vi "Create Cross Array.vi"() -> ()   [LabVIEW 2014]
uses:
  Slicer/LVslicer/Slice/TypeDefs/PowerSpeed.ctl
  Slicer/LVslicer/Slice/TypeDefs/PathSupreme.ctl
  Slicer/LVslicer/Slice/OverhangParam/PSup2SCAN/Sub/VelocityProfile.ctl
  Slicer/LVslicer/Slice/OverhangParam/PSup2SCAN/Sub/PathCut.ctl
  Slicer/LVslicer/Slice/OverhangParam/PSup2SCAN/Sub/Segment.ctl
  Slicer_11-28/LVslicer/Slice/TypeDefs/Point3D.ctl
  <vilib>/picture/3D Picture Control/Object/Create Object (name).vi
  <vilib>/picture/3D Picture Control/NI_3D Picture Control.lvlib
panel:
  out "Scale":cluster{dbl, dbl, dbl}
  in  "Spacing(mm)":dbl
  in  "Plate \nDiameter (mm)":dbl
  out "Stoped":bool
  in  "HighPower":dbl=500.0
  in  "Display":T1={"Mode"=enum."Inherit Value", "PointSize"=1.0, "LineWidth"=1.0}
  out "3D Picture":refnum<vi>(3d-picture)
  out "PathSupreme":T2
  in  "stop":bool
  in  "Create Array":bool
  in  "Create Cross":bool
  in  "Beam Width":dbl
  in  "# of Layers":dbl
  in  "Cross X dimension\n(cross is square)":dbl
  in  "HatchPower":T6={"Power"=300.0, "Mark Speed"=400.0, "Jump Speed"=1000.0}
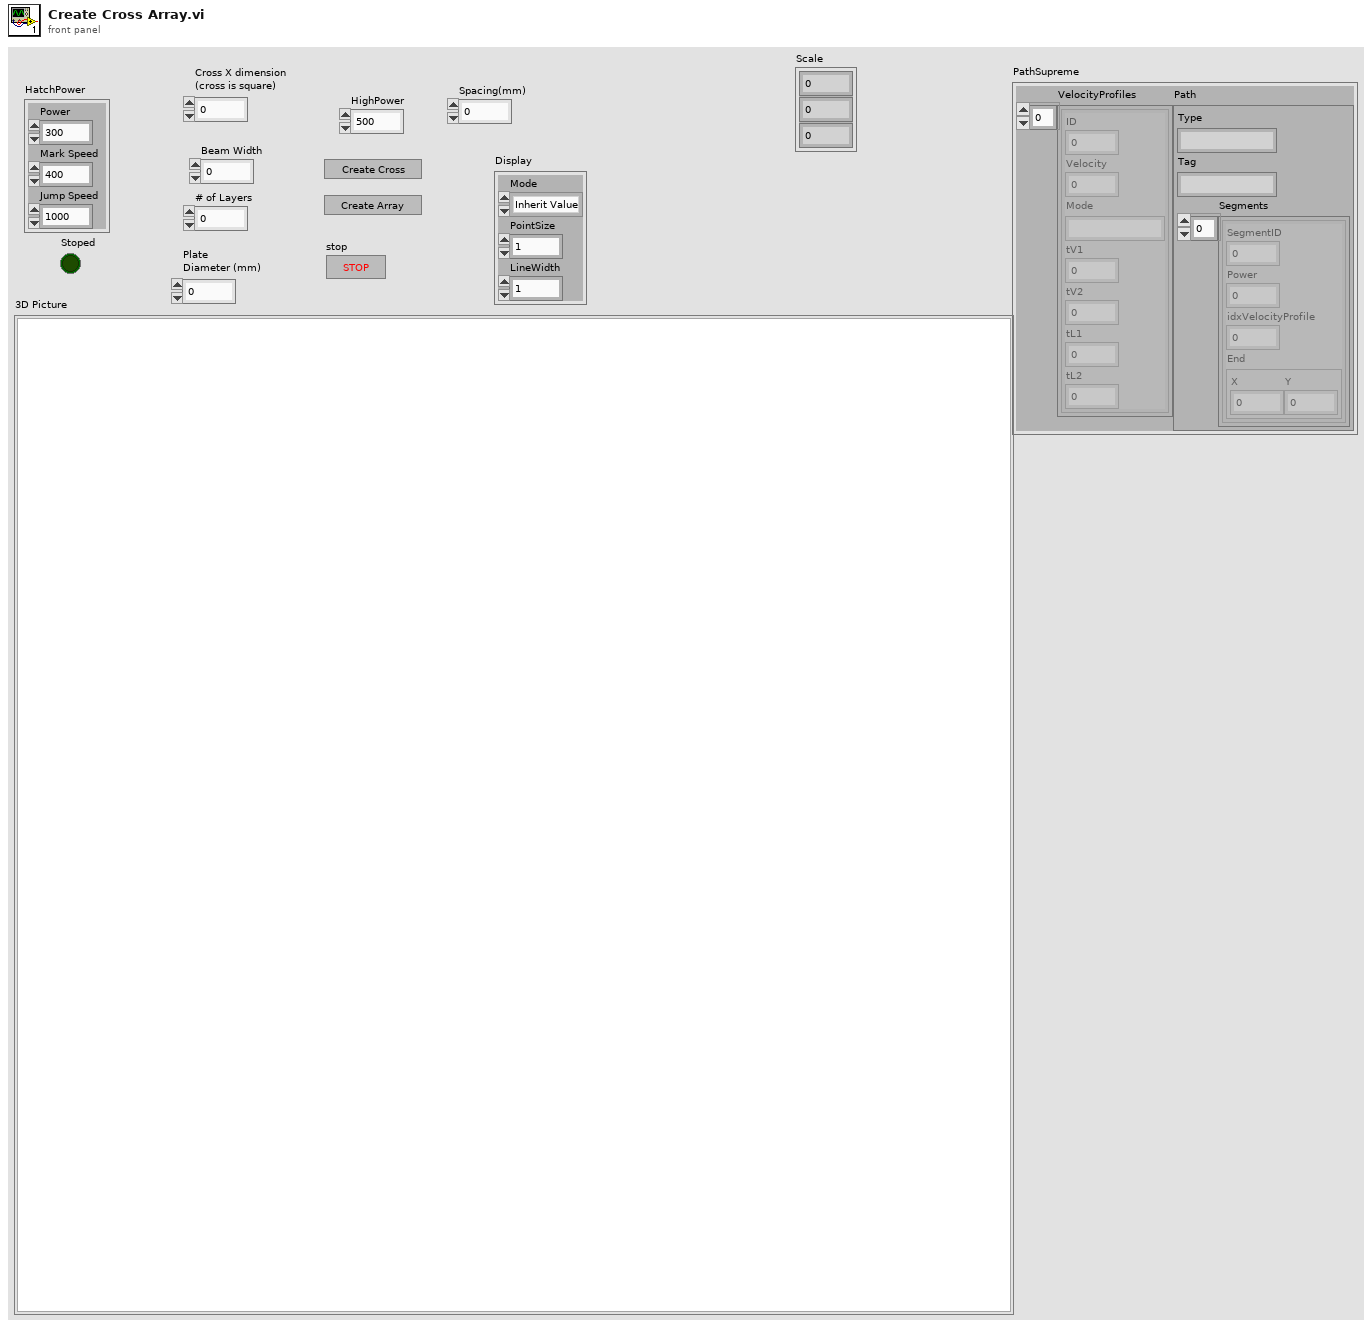
[diagram p1: front panel]
types:
  T1 = cluster{"Mode":enum16{"Inherit Value", "Points", "Wireframe", "Polygons"}, "PointSize":sgl, "LineWidth":sgl}
  T2 = typedef "PathSupreme.ctl" = cluster{"VelocityProfiles":T3[], "Path":T4}
  T3 = typedef "VelocityProfile.ctl" = cluster{"ID":u32, "Velocity":dbl, "Mode":string, "tV1":u32, "tV2":u32, "tL1":u32, "tL2":u32}
  T4 = typedef "PathCut.ctl" = cluster{"Type":string, "Tag":string, "Segments":T5[]}
  T5 = typedef "Segment.ctl" = cluster{"SegmentID":u16, "Power":sgl, "idxVelocityProfile":u16, "End":cluster{"X":sgl, "Y":sgl}}
  T6 = typedef "PowerSpeed.ctl" = cluster{"Power":dbl, "Mark Speed":dbl, "Jump Speed":dbl}
  T7 = enum16{"Idle", "Wait", "Create Cross", "Create Array", "Stop"}
  T8 = typedef "Point3D.ctl" = cluster{"X":sgl, "Y":sgl, "Z":sgl}
  T9 = cluster{"Lines":cluster{"P0":T8, "P1":T8}[], "Colors":u32[]}
  T10 = typedef "Point2DwSlope.ctl" = cluster{"X":sgl, "Y":sgl, "Slope":dbl}
  T11 = cluster{"VertexArray":T10[], "OnOffAr":enum16{"On", "Off"}[]}
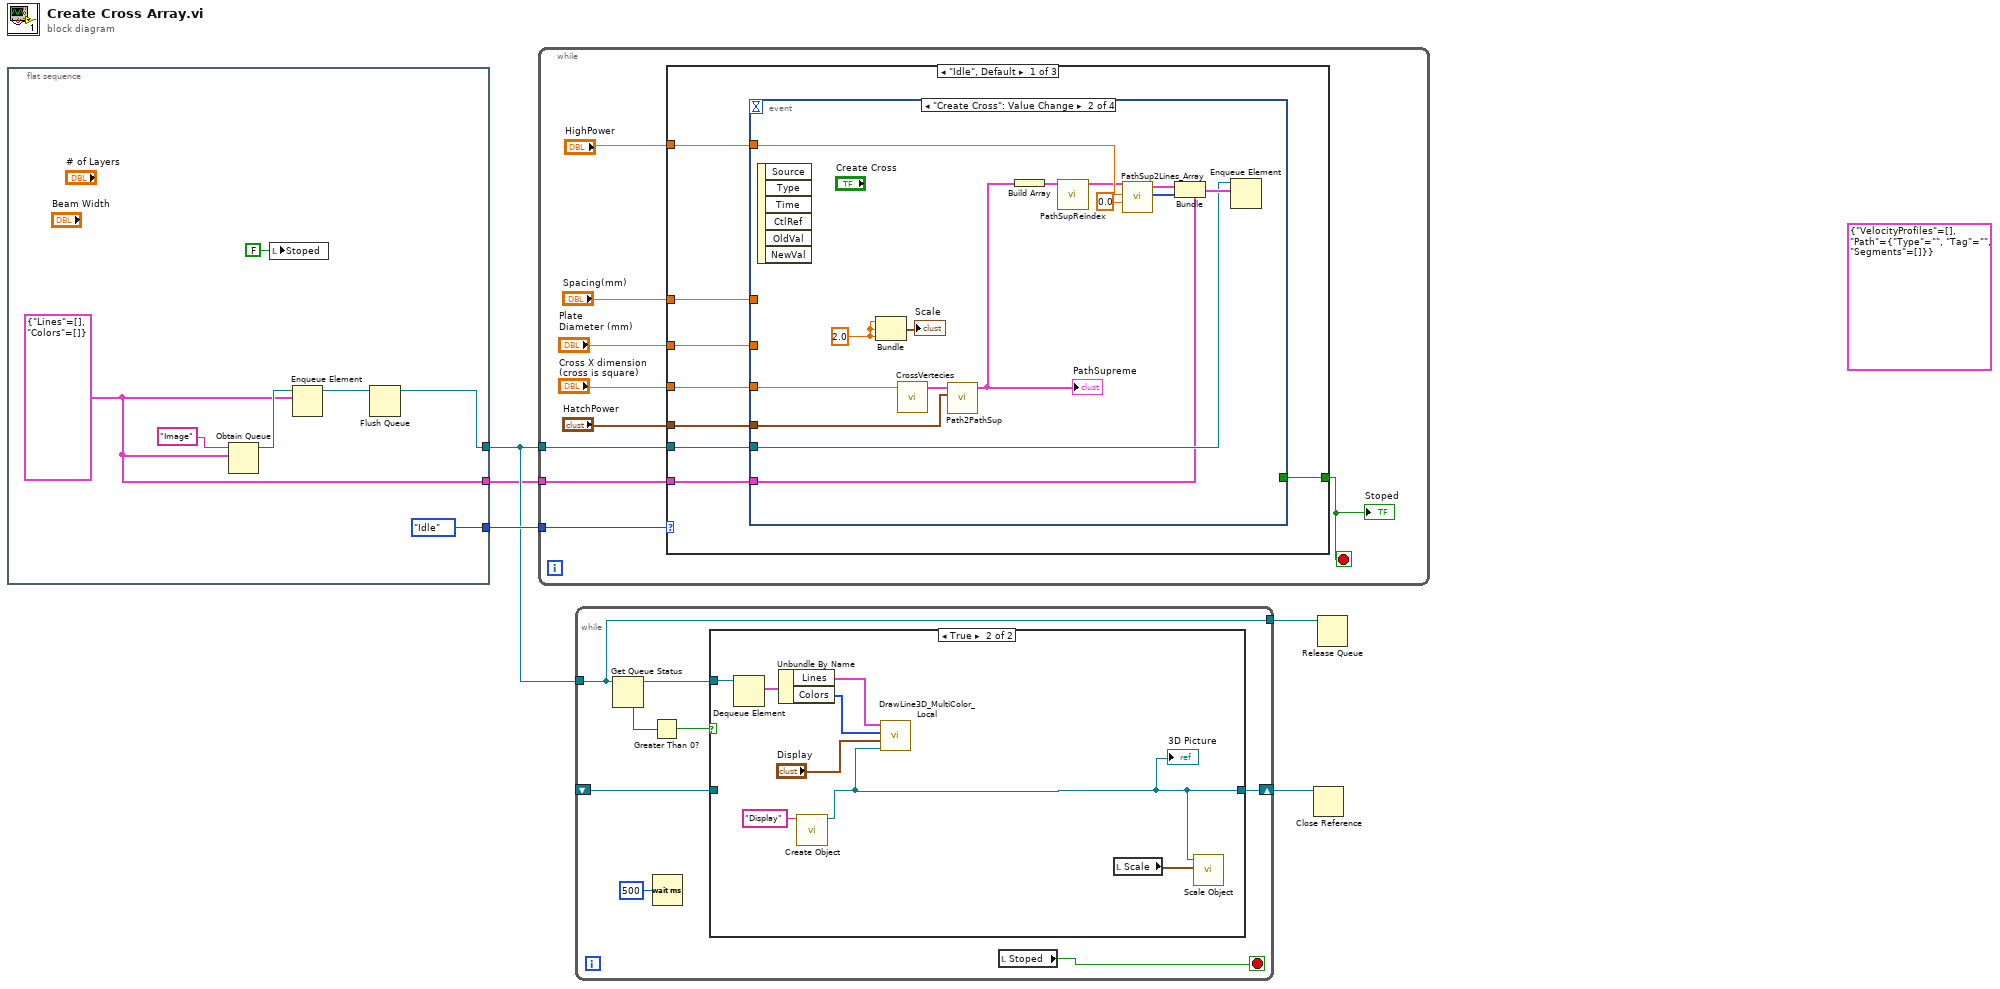
[diagram p0: block diagram]
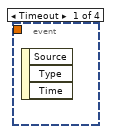
[diagram p2: hidden frame]
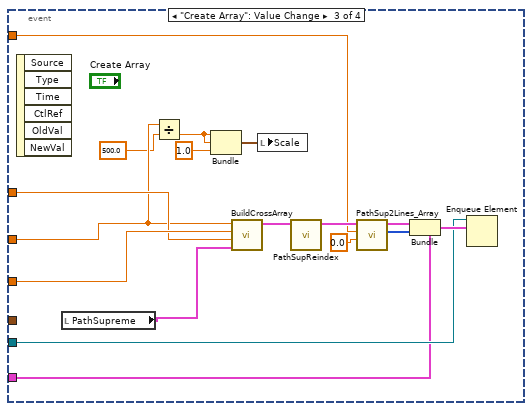
[diagram p3: hidden frame]
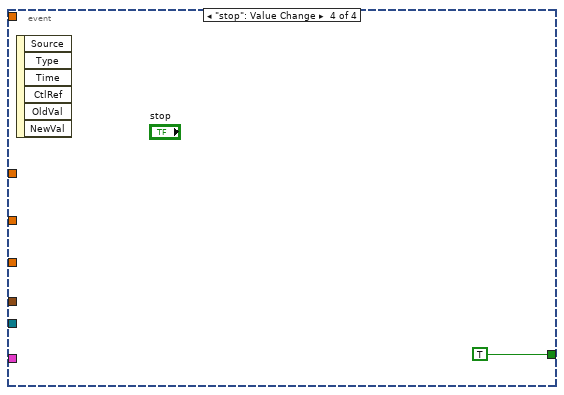
[diagram p4: hidden frame]
diagram:
  (unwired) T2 {"VelocityProfiles"=[], "Path"={"Type"="", "Tag"="", "Segments"=[]}} ("PathSupreme")
  n1 = flat-sequence {
    tunnel: [T7."Idle" ("Action")] -> w5
    tunnel: [w8] -> w4
    tunnel: [w7] -> w3
    frame #0 {
      w7 = T9 {"Lines"=[], "Colors"=[]} ("output cluster")
      n2 = Obtain Queue(name (unnamed)="Image", element data type=w7) -> (queue out=w10:refnum<queue>)  [unwired: 3 in, 2 out]
      n3 = local write "Stoped"(FALSE ("Stoped")) -> ()
      n4 = Enqueue Element(queue=w10, element=w7) -> (queue out=w9:refnum<queue>)  [unwired: 2 in, 2 out]
      n5 = Flush Queue(queue=w9) -> (queue out=w8:refnum<queue>)  [unwired: 1 in, 2 out]
    }
  }
  n6 = while {
    tunnel: w5 -> [w21]
    tunnel: w4 -> [w14]
    tunnel: w3 -> [w20]
    stop <- w19 stop-if-true
    n7 = case shown="\"Idle\", Default" w21 {
      tunnel: w14 -> [w29 _ _]
      tunnel: w20 -> [w28 _ _]
      tunnel: [w27 _ _] -> w19
      tunnel: "HighPower" -> [w26 _ _]
      tunnel: "Cross X dimension\n(cross is square)" -> [w25 _ _]
      tunnel: "HatchPower" -> [w24 _ _]
      tunnel: "Plate \nDiameter (mm)" -> [w23 _ _]
      tunnel: "Spacing(mm)" -> [w22 _ _]
      frame "Idle", Default {
        n8 = event shown="[1] \"Create Cross\": Value Change" {
          selector: _ -> [_ _ _ _]
          dyn-events: _ -> [_ _ _ _]
          timeout: _ -> [_ _ _ _]
          tunnel: w26 -> [_ w43 w52 _]
          tunnel: w29 -> [_ w36 w51 _]
          tunnel: w28 -> [_ w35 w50 _]
          tunnel: [_ _ _ TRUE] -> w27
          tunnel: w25 -> [_ w33 w61 _]
          tunnel: w24 -> [_ w32 _ _]
          tunnel: w23 -> [_ _ w46 _]
          tunnel: w22 -> [_ _ w60 _]
          event Timeout {
            n9 = event-data() -> ()  [unwired: 1 in, 3 out]
          }
          event "Create Cross": Value Change {
            w31 = 2.0
            n10 = event-data() -> ()  [unwired: 1 in, 6 out]
            n11 = Bundle(w31, w31, w31) -> (→"Scale":cluster{dbl, dbl, dbl})  [unwired: 1 in]
            n12 = call "CrossVertecies.vi"("Cross X dimension\n(cross is square)"=w33) -> ("Combined"=w44:T11)  [unwired: 4 in]
            n13 = call "Path2PathSup.vi"("PowerSpeed"=w32, "Combined"=w44) -> ("PathSupreme"=w34:T2)  [unwired: 9 in]
            "PathSupreme" <- w34
            n14 = Build Array(w34) -> (w40:T2[])
            n15 = call "PathSupReindex.vi"("PathSupremes"=w40) -> ("PathSupOut"=w41:T2[])  [unwired: 10 in]
            n16 = call "PathSup2Lines_Array.vi"("Z"=0.0, "HighPower"=w43, "PathSupIn"=w41) -> ("Colors"=w38:u32[], "Lines"=w39:cluster{"P0":T8, "P1":T8}[])  [unwired: 7 in]
            n17 = Bundle(cluster=w35, "Lines"=w39, "Colors"=w38) -> (w37:T9)
            n18 = Enqueue Element(queue=w36, element=w37) -> ()  [unwired: 2 in, 3 out]
          }
          event "Create Array": Value Change {
            n19 = event-data() -> ()  [unwired: 1 in, 6 out]
            n20 = local read "PathSupreme"() -> (w59:T2)
            n21 = Divide(x=w46, y=500.0 ("x")) -> (x/y=w47:dbl)
            n22 = Bundle(w47, w47, 1.0) -> (w48:cluster{dbl, dbl, dbl})  [unwired: 1 in]
            n23 = call "BuildCrossArray.vi"("Plate \nDiameter (mm)"=w46, "Cross X dimension\n(cross is square)"=w61, "Desired\nSpacing(mm)"=w60, "PathSupreme"=w59) -> ("PathSupreams"=w53:T2[])  [unwired: 3 in, 1 out]
            n24 = local write "Scale"(w48) -> ()
            n25 = call "PathSupReindex.vi"("PathSupremes"=w53) -> ("PathSupOut"=w57:T2[])  [unwired: 10 in]
            n26 = call "PathSup2Lines_Array.vi"("Z"=0.0, "HighPower"=w52, "PathSupIn"=w57) -> ("Colors"=w55:u32[], "Lines"=w56:cluster{"P0":T8, "P1":T8}[])  [unwired: 7 in]
            n27 = Bundle(cluster=w50, "Lines"=w56, "Colors"=w55) -> (w54:T9)
            n28 = Enqueue Element(queue=w51, element=w54) -> ()  [unwired: 2 in, 3 out]
          }
          event "stop": Value Change {
            n29 = event-data() -> ()  [unwired: 1 in, 6 out]
          }
        }
      }
      frame "Wait" {
      }
      frame "Create Cross" {
      }
    }
    "Stoped" <- w19
  }
  n30 = while {
    tunnel: w4 -> [w66]
    tunnel: [w66] -> w1
    shift-right: [w64] -> w2
    shift-left: _ -> [w63]
    stop <- w65 stop-if-true
    n31 = Get Queue Status(queue=w66) -> (queue out=w69:refnum<queue>, # elements in queue=w68:i32)  [unwired: 2 in, 6 out]
    n32 = Greater Than 0?(x=w68) -> (x > 0?=w67:bool)
    n33 = Wait (ms)(milliseconds to wait=u32 500) -> ()  [unwired: 1 out]
    n34 = case shown="True" w67 {
      tunnel: w69 -> [_ w78]
      tunnel: [w71 w72] -> w64
      tunnel: w63 -> [w71 _]
      frame False {
      }
      frame True {
        n35 = Dequeue Element(queue=w78) -> (element=w77:T9)  [unwired: 2 in, 3 out]
        n36 = Unbundle By Name(w77) -> ("Lines"=w76:cluster{"P0":T8, "P1":T8}[], "Colors"=w75:u32[])
        n37 = call-poly <vilib>:"Create Object.vi"("Name"="Display") -> ("Scene:New Object"=w72:refnum<vi>)  [unwired: 9 in, 1 out]
        "3D Picture" <- w72
        n38 = call "DrawLine3D_MultiColor_Local.vi"("Scene Object In"=w72, "Display"="Display", "Colors"=w75, "Lines"=w76) -> ()  [unwired: 7 in, 1 out]
        n39 = local read "Scale"() -> (w73:cluster{dbl, dbl, dbl})
        n40 = call <vilib>:"Scale Object.vi"("Scale"=w73, "Scene.Object In"=w72) -> ()  [unwired: 8 in, 2 out]
      }
    }
    n41 = local read "Stoped"() -> (w65:bool)
  }
  n42 = Close Reference(reference=w2) -> ()  [unwired: 1 in, 1 out]
  n43 = Release Queue(queue=w1) -> ()  [unwired: 2 in, 3 out]
